vi "Read Device Name.vi"(8 "error in (no error)":errorcluster, 11 "PLBB in":refnum<class "PL BlackBox Modbus Client.lvclass">) -> (0 "error out":errorcluster, 2 "device name":string, 3 "PLBB out":refnum<class "PL BlackBox Modbus Client.lvclass">)   [LabVIEW 2015, in "PL BlackBox Modbus Client.lvclass"]
doc: "Reads the device name."
uses:
  PL BlackBox Modbus Client.lvclass
  <vilib>/plasmapper/PL Modbus Client/PL Modbus Client.lvclass
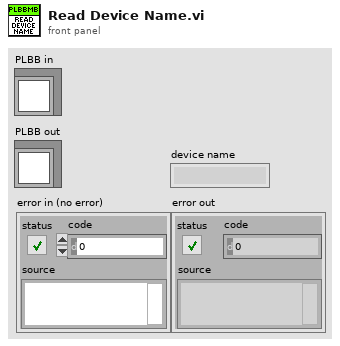
[diagram p1: front panel]
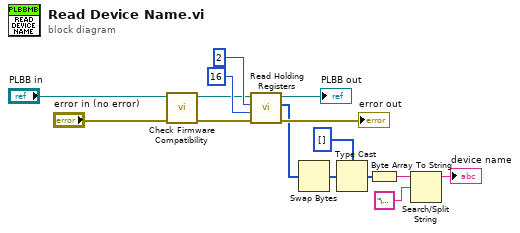
[diagram p0: block diagram]
diagram:
  n1 = call-dynamic "Check Firmware Compatibility.vi"("error in (no error)"="error in (no error)", "PLBB in"="PLBB in") -> ("error out"=w2:errorcluster, "PLBB out"=w1:refnum<class "PL BlackBox Modbus Client.lvclass">)  [unwired: 8 in]
  n2 = call <vilib>:"Read Holding Registers.vi"("error in (no error)"=w2, "number of holding registers"=u16 16 ("address"), "address"=u16 2, "MODBUS in"=w1) -> ("error out"=→"error out":errorcluster, "values"=w6:u16[], "MODBUS out"=→"PLBB out":refnum<class "PL BlackBox Modbus Client.lvclass">)  [unwired: 5 in]
  n3 = Swap Bytes(anything=w6) -> (byte swapped=w9:u16[])
  n4 = Type Cast(type=u8[] [] ("values"), x=w9) -> (*(type *) &x=w11:u8[])
  n5 = Byte Array To String(unsigned byte array=w11) -> (string=w8:string)
  n6 = Search/Split String(string=w8, search string/char (-)="\u0000") -> (substring before match=→"device name":string)  [unwired: 1 in, 2 out]
